vi "Process to IO.vi"(8 "error in":errorcluster, 11 "Process in":T1) -> (0 "error out":errorcluster, 3 "Process out":T2)   [LabVIEW 2019, in "Fluidic Process.lvlib"]
uses:
  Fluidic Process.lvlib
  IO/sbRIO9623/SubVI/IO Control.ctl
  Fluidic Data.ctl
  IO/sbRIO9623/sbRIO9623.lvlib
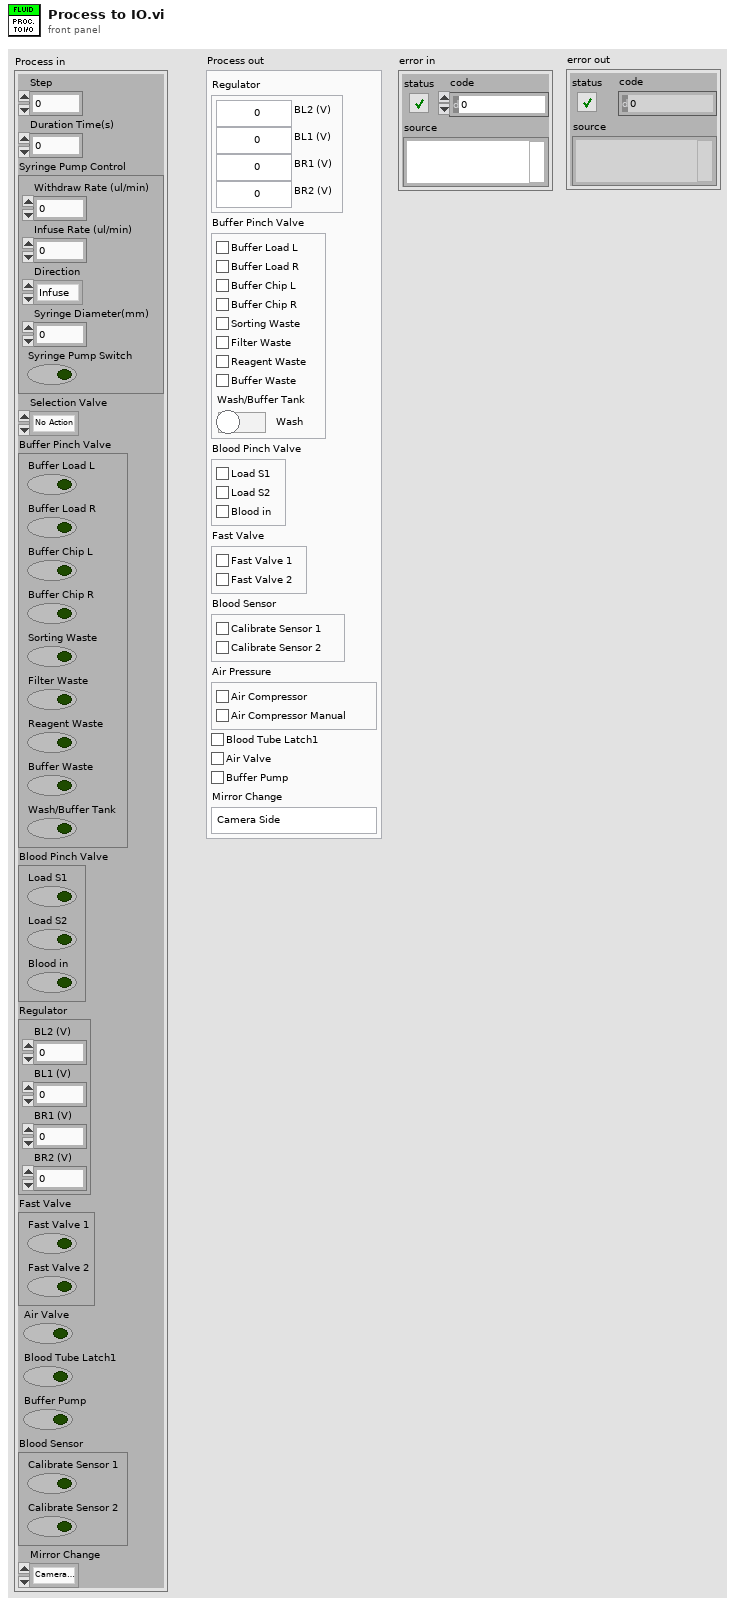
[diagram p1: front panel]
types:
  T1 = typedef "Fluidic Process.lvlib/Fluidic Data.ctl" = cluster{"Step":i32, "Duration Time(s)":i32, "Syringe Pump Control":cluster{"Withdraw Rate (ul/min)":dbl, "Infuse Rate (ul/min)":dbl, "Direction":enum16{"Infuse", "Withdraw"}, "Syringe Diameter(mm)":dbl, "Syringe Pump Switch":bool}, "Selection Valve":enum16{"No Action", "Position 1", "Position 2", "Position 3", "Position 4", "Position 5", "Position 6"}, "Buffer Pinch Valve":cluster{"Buffer Load L":bool, "Buffer Load R":bool, "Buffer Chip L":bool, "Buffer Chip R":bool, "Sorting Waste":bool, "Filter Waste":bool, "Reagent Waste":bool, "Buffer Waste":bool, "Wash/Buffer Tank":bool}, "Blood Pinch Valve":cluster{"Load S1":bool, "Load S2":bool, "Blood in":bool}, "Regulator":cluster{"BL2 (V)":fxp<+,16,3>, "BL1 (V)":fxp<+,16,3>, "BR1 (V)":fxp<+,16,3>, "BR2 (V)":fxp<+,16,3>}, "Fast Valve":cluster{"Fast Valve 1":bool, "Fast Valve 2":bool}, "Air Valve":bool, "Blood Tube Latch1":bool, "Buffer Pump":bool, "Blood Sensor":cluster{"Calibrate Sensor 1":bool, "Calibrate Sensor 2":bool}, "Mirror Change":enum16{"Camera Side", "SiPM Side"}}
  T2 = typedef "sbRIO9623.lvlib/IO Control.ctl" = cluster{"Regulator":cluster{"BL2 (V)":fxp<+,16,3>, "BL1 (V)":fxp<+,16,3>, "BR1 (V)":fxp<+,16,3>, "BR2 (V)":fxp<+,16,3>}, "Buffer Pinch Valve":cluster{"Buffer Load L":bool, "Buffer Load R":bool, "Buffer Chip L":bool, "Buffer Chip R":bool, "Sorting Waste":bool, "Filter Waste":bool, "Reagent Waste":bool, "Buffer Waste":bool, "Wash/Buffer Tank":bool}, "Blood Pinch Valve":cluster{"Load S1":bool, "Load S2":bool, "Blood in":bool}, "Fast Valve":cluster{"Fast Valve 1":bool, "Fast Valve 2":bool}, "Blood Sensor":cluster{"Calibrate Sensor 1":bool, "Calibrate Sensor 2":bool}, "Air Pressure":cluster{"Air Compressor":bool, "Air Compressor Manual":bool}, "Blood Tube Latch1":bool, "Air Valve":bool, "Buffer Pump":bool, "Mirror Change":enum16{"Camera Side", "SiPM Side"}}
  T3 = cluster{"Air Compressor":bool, "Air Compressor Manual":bool}
  T4 = cluster{"BL2 (V)":fxp<+,16,3>, "BL1 (V)":fxp<+,16,3>, "BR1 (V)":fxp<+,16,3>, "BR2 (V)":fxp<+,16,3>}
  T5 = cluster{"Buffer Load L":bool, "Buffer Load R":bool, "Buffer Chip L":bool, "Buffer Chip R":bool, "Sorting Waste":bool, "Filter Waste":bool, "Reagent Waste":bool, "Buffer Waste":bool, "Wash/Buffer Tank":bool}
  T6 = cluster{"Load S1":bool, "Load S2":bool, "Blood in":bool}
  T7 = cluster{"Fast Valve 1":bool, "Fast Valve 2":bool}
  T8 = cluster{"Calibrate Sensor 1":bool, "Calibrate Sensor 2":bool}
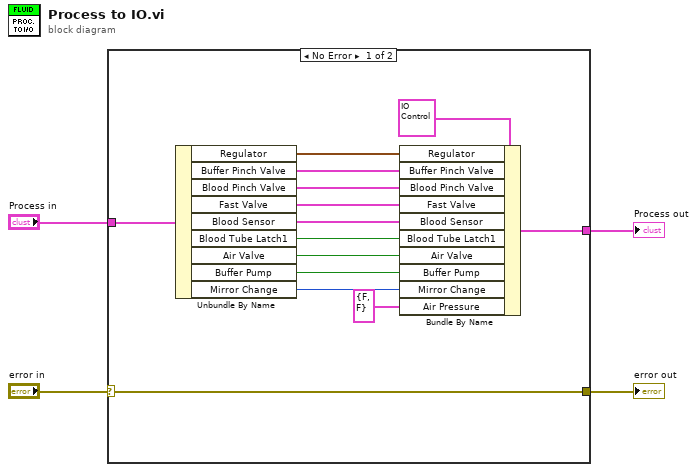
[diagram p0: block diagram]
diagram:
  n1 = case shown="No Error" "error in" {
    selector: "error in" -> [w5 w19]
    tunnel: "Process in" -> [w18 _]
    tunnel: [w6 _] -> w3
    tunnel: [w5 w19] -> w1
    frame No Error {
      n2 = Unbundle By Name(w18) -> ("Regulator"=w16:T4, "Buffer Pinch Valve"=w15:T5, "Blood Pinch Valve"=w14:T6, "Fast Valve"=w13:T7, "Blood Sensor"=w12:T8, "Blood Tube Latch1"=w11:bool, "Air Valve"=w10:bool, "Buffer Pump"=w9:bool, "Mirror Change"=w8:enum16{"Camera Side", "SiPM Side"})
      n3 = Bundle By Name(cluster=T2 {"Regulator"={"BL2 (V)"=0.0, "BL1 (V)"=0.0, "BR1 (V)"=0.0, "BR2 (V)"=0.0}, "Buffer Pinch Valve"={"Buffer Load L"=FALSE, "Buffer Load R"=FALSE, "Buffer Chip L"=FALSE, "Buffer Chip R"=FALSE, "Sorting Waste"=FALSE, "Filter Waste"=FALSE, "Reagent Waste"=FALSE, "Buffer Waste"=FALSE, "Wash/Buffer Tank"=FALSE}, "Blood Pinch Valve"={"Load S1"=FALSE, "Load S2"=FALSE, "Blood in"=FALSE}, "Fast Valve"={"Fast Valve 1"=FALSE, "Fast Valve 2"=FALSE}, "Blood Sensor"={"Calibrate Sensor 1"=FALSE, "Calibrate Sensor 2"=FALSE}, "Air Pressure"={"Air Compressor"=FALSE, "Air Compressor Manual"=FALSE}, "Blood Tube Latch1"=FALSE, "Air Valve"=FALSE, "Buffer Pump"=FALSE, "Mirror Change"=enum."Camera Side"} ("I/O Control"), "Regulator"=w16, "Buffer Pinch Valve"=w15, "Blood Pinch Valve"=w14, "Fast Valve"=w13, "Blood Sensor"=w12, "Blood Tube Latch1"=w11, "Air Valve"=w10, "Buffer Pump"=w9, "Mirror Change"=w8, "Air Pressure"=T3 {"Air Compressor"=FALSE, "Air Compressor Manual"=FALSE}) -> (w6:T2)
    }
    frame Error {
    }
  }
  "Process out" <- w3
  "error out" <- w1
